vi "Drive Encoders.vi"(1 "Inversions":bool[](array[boolean]), 2 "Reset":bool, 3 "Mode":enum8{"Start", "Run", "Finish"}(ring)) -> (0 "Encoder":T1(array[cluster]))   [LabVIEW 2014]
uses:
  <vilib>/Rock Robotics/WPI/CAN/TalonSRX/WPI_CANTalonSRX_APIFeedbackSelect.ctl
  <vilib>/Analysis/2dsp.llb/Integral Method.ctl
  Precreated VIs/Robot Global Data.vi
  <vilib>/Analysis/NI_AALPro.lvlib
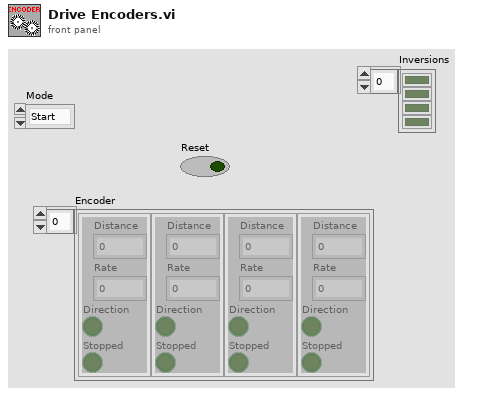
[diagram p1: front panel]
types:
  T1 = cluster{"Distance":dbl, "Rate":dbl, "Direction":bool, "Stopped":bool}[]
  T2 = typedef "WPI_CANTalonSRX_APIFeedbackSelect.ctl" = enum16{"Digital Quadrature Encoder", "Analog Potentiometer", "Analog Encoder"}
  T3 = typedef "WPI_MotorControlDeviceRef.ctl" = cluster{"DeviceStatus":errorcluster, "Type":T4, "PWM":cluster{"Controller":T5, "PWM Channel":T6, "DeadBand":T7}, "CAN":cluster{"Device Number":u8, "Control Mode":T8, "Semaphore":T9, "Max Vout":dbl, "TalonSRX Control Mode":T10}, "Invert":bool, "TransformRef":T11, "InvTransformRef":T11}
  T4 = typedef "WPI_MotorControlType.ctl" = enum16{"PWM", "CAN", "CANTalonSRX"}
  T5 = typedef "FPGA_TypedefDigitalModule.ctl" = enum16{"Controller 1"}
  T6 = typedef "FPGA_DIOPWMChannel.ctl" = enum8{"PWM 0", "PWM 1", "PWM 2", "PWM 3", "PWM 4", "PWM 5", "PWM 6", "PWM 7", "PWM 8", "PWM 9", "PWM MXP 0", "PWM MXP 1", "PWM MXP 2", "PWM MXP 3", "PWM MXP 4", "PWM MXP 5", "PWM MXP 6", "PWM MXP 7", "PWM MXP 8", "PWM MXP 9", "Invalid"}
  T7 = typedef "WPI_PWMDeadband.ctl" = cluster{"Name":string, "maxPositivePwm":i32, "minPositivePwm":i32, "centerPwm":i32, "maxNegativePwm":i32, "minNegativePwm":i32, "angularRange":u16}
  T8 = typedef "WPI_CANJaguar_ControlMode.ctl" = enum8{"Percent VBus", "Current", "Speed", "Position", "Voltage"}
  T9 = typedef "Semaphore RefNum" = refnum<k1>
  T10 = typedef "WPI_CANTalonSRX_APIControlMode.ctl" = enum8{"Percent VBus", "Speed", "Position", "Slave", "Unchanged / Invalid"}
  T11 = typedef "WPI_PWMTransform_ConPane.ctl" = refnum<vi>
  T12 = typedef "NI_AALPro.lvlib/Integral Method.ctl" = i32
  T13 = typedef "WPI_CANTalonSRX_GlobalStatus.ctl" = cluster{"Applied Throttle":dbl, "Module Enabled":bool, "CAN Error":errorcluster, "Closed Loop Error":dbl, "Forward Limit Switch Closed":bool, "Reverse Limit Switch Closed":bool, "Sensor Position":dbl, "Sensor Velocity":dbl, "Current":dbl, "Sticky Fault - Over Temp":bool, "Sticky Fault - Under Voltage":bool, "Sticky Fault - Forward Limit":bool, "Sticky Fault - Reverse Limit":bool, "Sticky Fault - Forward Soft Limit":bool, "Sticky Fault - Reverse Soft Limit":bool, "Brake is Enabled":bool, "Encoder Position":dbl, "Encoder Velocity":dbl, "Encoder Index Count":dbl, "Encoder A Pin State":bool, "Encoder B Pin State":bool, "Encoder Index Pin State":bool, "Analog In":dbl, "Analog In Velocity":dbl, "Temperature (C)":dbl, "Battery Voltage":dbl}
  T14 = cluster{"Distance":dbl, "Rate":dbl, "Direction":bool, "Stopped":bool}
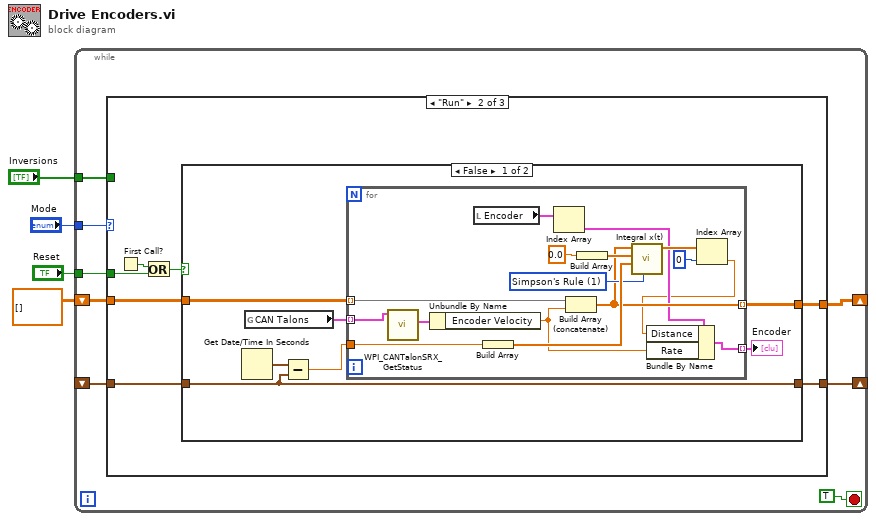
[diagram p0: block diagram]
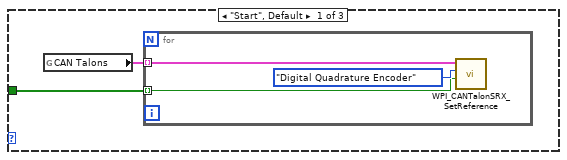
[diagram p2: hidden frame]
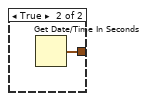
[diagram p3: hidden frame]
diagram:
  n1 = while {
    tunnel: "Mode" -> [w12]
    tunnel: "Reset" -> [w10]
    tunnel: "Inversions" -> [w9]
    shift-right: [w8] -> _
    shift-left: _ -> [w7]
    shift-right: [w6] -> _
    shift-left: dbl[][] [] -> [w5]
    stop <- TRUE stop-if-true
    n2 = case shown="\"Run\"" w12 {
      tunnel: w10 -> [_ w24 _]
      tunnel: w9 -> [w13 _ _]
      tunnel: [_ w23 _] -> w8
      tunnel: w7 -> [_ w20 _]
      tunnel: [_ w19 _] -> w6
      tunnel: w5 -> [_ w18 _]
      frame "Start", Default {
        n3 = global read "Robot Global Data.vi" "CAN Talons"() -> (w14:T3[])
        n4 = for {
          tunnel: w14 -> [w17] mode=indexing
          tunnel: w13 -> [w15] mode=indexing
          n5 = call <vilib>:"WPI_CANTalonSRX_SetReference.vi"("Reverse Feedback Sensor"=w15, "Feedback Reference"=WPI_CANTalonSRX_APIFeedbackSelect."Digital Quadrature Encoder", "CAN Talon SRX Ref"=w17) -> ()  [unwired: 7 in, 2 out]
        }
      }
      frame "Run" {
        n6 = First Call?() -> (First Call?: T/F=w21:bool)
        n7 = Or(x=w21, y=w24) -> (x .or. y?=w22:bool)
        n8 = case shown="False" w22 {
          tunnel: [w29 w48] -> w23
          tunnel: w20 -> [w29 _]
          tunnel: [w27 _] -> w19
          tunnel: w18 -> [w26 _]
          frame False {
            n9 = Get Date/Time In Seconds() -> (seconds since 1Jan1904=w28:timestamp)
            n10 = global read "Robot Global Data.vi" "CAN Talons"() -> (w31:T3[])
            n11 = Subtract(x=w28, y=w29) -> (x-y=w30:dbl)
            n12 = for {
              tunnel: w31 -> [w47] mode=indexing
              tunnel: w30 -> [w42]
              tunnel: [w37] -> w27 mode=indexing
              tunnel: w26 -> [w36] mode=indexing
              tunnel: [w32] -> w25 mode=indexing
              w40 = T12 1 items=["Trapezoidal Rule", "Simpson's Rule", "Simpson's 3/8 Rule", "Bode Rule"] ("integration method")
              n13 = call <vilib>:"WPI_CANTalonSRX_GetStatus.vi"("CAN Talon SRX Ref"=w47) -> ("Talon SRX Status"=w45:T13)  [unwired: 8 in, 2 out]
              n14 = Unbundle By Name(w45) -> ("Encoder Velocity"=w34:dbl)
              n15 = local read "Encoder"() -> (w46:T1)
              n16 = Build Array(w42) -> (w41:dbl[])
              n17 = Index Array(array=w46) -> (element=w35:T14)  [unwired: 1 in]
              n18 = Build Array (concatenate)(w36, w34) -> (w37:dbl[])
              n19 = Build Array(0.0 ("element")) -> (w44:dbl[])
              n20 = call <vilib>:"Integral x(t).vi"("integration method"=w40, "Final Condition"=w41, "Initial Condition"=w44, "X"=w37) -> ("Integral X"=w39:dbl[])  [unwired: 6 in, 1 out]
              n21 = Index Array(array=w39, index=0) -> (element=w33:dbl)
              n22 = Bundle By Name(cluster=w35, "Distance"=w33, "Rate"=w34) -> (w32:T14)
            }
            "Encoder" <- w25
          }
          frame True {
            n23 = Get Date/Time In Seconds() -> (seconds since 1Jan1904=w48:timestamp)
          }
        }
      }
      frame "Finish" {
      }
    }
  }
